vi "Spartan Test.vi"() -> ()   [LabVIEW 2011]
panel:
  out "DIAdem Desktop Folder":path
  out "blink":bool
  in  "stop":bool
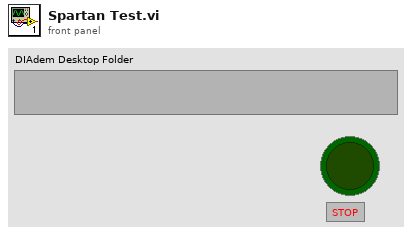
[diagram p1: front panel]
types:
  T1 = typedef "DIAdem Reference.ctl" = cluster{"ToCommand Reference":refnum<k7>, "ToDataSheet Reference":refnum<k7>}
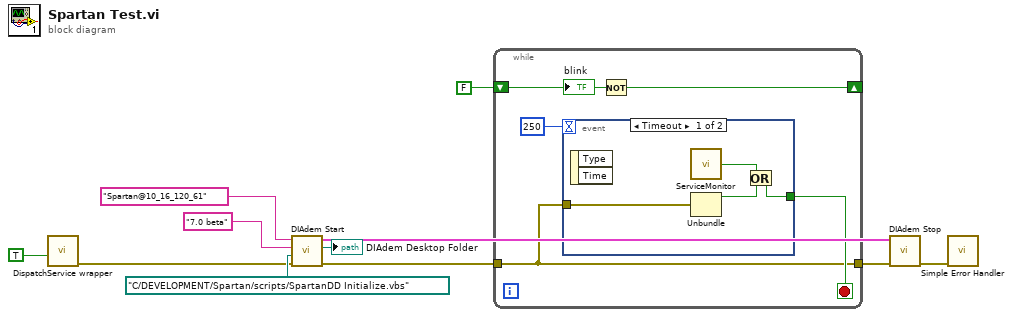
[diagram p0: block diagram]
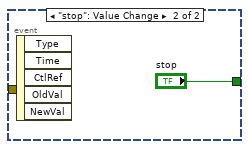
[diagram p2: hidden frame]
diagram:
  n1 = call "DispatchService wrapper.vi"("Dispatch Service? (f)"=TRUE) -> ("error out"=w2:errorcluster)  [unwired: 1 in, 9 out]
  n2 = call "DIAdem Start.vi"("error in"=w2, "Init VBS Full Path (empty)"=path "C:/DEVELOPMENT/Spartan/scripts/SpartanDD Initialize.vbs", "Version String (\"\")"="7.0 beta" ("DataFinder (\"\")"), "DataFinder (\"\")"="Spartan@10_16_120_61" ("DataFinder (\"\")")) -> ("error out"=w10:errorcluster, "DIAdem Desktop File"=→"DIAdem Desktop Folder":path, "DIAdem Reference"=w8:T1)  [unwired: 5 in]
  n3 = while {
    shift-right: [w13] -> _
    shift-left: FALSE -> [w14]
    tunnel: w10 -> [w12]
    tunnel: [w12] -> w9
    stop <- w16 stop-if-true
    n4 = event shown="[0] Timeout" {
      selector: _ -> [_ _]
      dyn-events: _ -> [_ _]
      timeout: 250 -> [_ _]
      tunnel: [w18 "stop"] -> w16
      tunnel: w12 -> [w20 _]
      event Timeout {
        n5 = event-data() -> ()  [unwired: 1 in, 2 out]
        n6 = call "ServiceMonitor.vi"() -> ("Stop?"=w17:bool)  [unwired: 1 in]
        n7 = Unbundle(w20) -> ("status"=w19:bool)  [unwired: 2 out]
        n8 = Or(x=w17, y=w19) -> (x .or. y?=w18:bool)
      }
      event "stop": Value Change {
        n9 = event-data() -> ()  [unwired: 1 in, 5 out]
      }
    }
    n10 = Not(x=w14) -> (.not. x?=w13:bool)
    "blink" <- w14
  }
  n11 = call "DIAdem Stop.vi"("error in (no error)"=w9, "DIAdem Reference"=w8) -> ("error out"=w7:errorcluster)  [unwired: 6 in]
  n12 = call <vilib>:"Simple Error Handler.vi"("error in (no error)"=w7) -> ()  [unwired: 4 in, 5 out]
